vi "Check_alarm.vi"(0 "Data_Control":T1={"Lavatory_A"={"Timer"=timestamp(0 s since 1904-01-01), "Occupied"=FALSE}, "Lavatory_B"={"Timer"=timestamp(0 s since 1904-01-01), "Occupied"=FALSE}, "Lavatory_C"={"Timer"=timestamp(0 s since 1904-01-01), "Occupied"=FALSE}, "Lavatory_D"={"Timer"=timestamp(0 s since 1904-01-01), "Occupied"=FALSE}, "Seat_belt"=TRUE, "Alarm"=TRUE, "Lavatory"="", "Timr_Limit"=0, "Time_Now"=timestamp(0 s since 1904-01-01)}) -> (4 "Trigger A":bool, 6 "Trigger B":bool, 8 "Trigger C":bool, 10 "Trigger D":bool)   [LabVIEW 2023, in "Lavatory_Management.lvlib"]
uses:
  Lavatory_Management.lvlib
  Controls/Managemet_data.ctl
  Controls/Lavatory_data.ctl
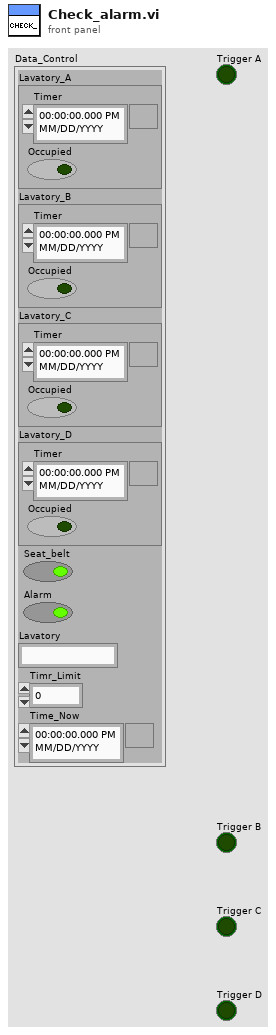
[diagram p1: front panel]
types:
  T1 = typedef "Lavatory_Management.lvlib/Managemet_data.ctl" = cluster{"Lavatory_A":T2, "Lavatory_B":T2, "Lavatory_C":T2, "Lavatory_D":T2, "Seat_belt":bool, "Alarm":bool, "Lavatory":string, "Timr_Limit":i32, "Time_Now":timestamp}
  T2 = typedef "Lavatory_Management.lvlib/Lavatory_data.ctl" = cluster{"Timer":timestamp, "Occupied":bool}
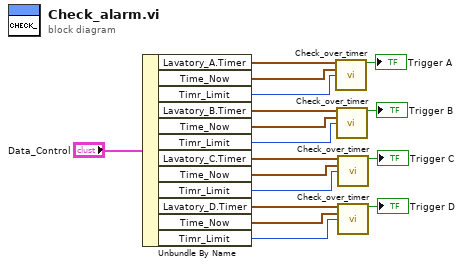
[diagram p0: block diagram]
diagram:
  n1 = Unbundle By Name("Data_Control") -> ("Lavatory_A.Timer"=w16:timestamp, "Time_Now"=w15:timestamp, "Timr_Limit"=w14:i32, "Lavatory_B.Timer"=w13:timestamp, "Time_Now"=w12:timestamp, "Timr_Limit"=w11:i32, "Lavatory_C.Timer"=w10:timestamp, "Time_Now"=w9:timestamp, "Timr_Limit"=w8:i32, "Lavatory_D.Timer"=w7:timestamp, "Time_Now"=w6:timestamp, "Timr_Limit"=w5:i32)
  n2 = call "Check_over_timer.vi"("Lavatory TImer"=w16, "Time Now"=w15, "Limit"=w14) -> ("Trigger"=→"Trigger A":bool)  [unwired: 12 in]
  n3 = call "Check_over_timer.vi"("Lavatory TImer"=w13, "Time Now"=w12, "Limit"=w11) -> ("Trigger"=→"Trigger B":bool)  [unwired: 12 in]
  n4 = call "Check_over_timer.vi"("Lavatory TImer"=w10, "Time Now"=w9, "Limit"=w8) -> ("Trigger"=→"Trigger C":bool)  [unwired: 12 in]
  n5 = call "Check_over_timer.vi"("Lavatory TImer"=w7, "Time Now"=w6, "Limit"=w5) -> ("Trigger"=→"Trigger D":bool)  [unwired: 12 in]
